vi "Encode Channels.vi"(8 "error in":errorcluster, 10 "Data and Parameters":T2 {"Data" format="%.0b"}, 11 "Values in":dbl[](array[numeric])) -> (0 "error out":errorcluster, 3 "Data":u8[](array[numeric]) format="%.0b")   [LabVIEW 2020, in "AIM ARINC 664 Engine.lvlib" / "Implementation.lvlib" / "Tx UDP Execution Unit.lvclass"]
uses:
  Tx UDP Execution Unit.lvclass
  <vilib>/NI/NI VeriStand Encoding and Decoding/Encoding.ctl
  b24d3698-aaae-4200-bf93-4b6af5480478.vi
  5b1080be-549e-4688-aad8-fb955257d8ef.vi
  b24d3698-aaae-4200-bf93-4b6af5480478.vi/9377bb8f-44b5-4a8f-87f1-966fd5a9edcc.vi
  b24d3698-aaae-4200-bf93-4b6af5480478.vi/e95d9d1f-307c-44d6-9f26-c3f519a4990d.vi
  b24d3698-aaae-4200-bf93-4b6af5480478.vi/0c23f515-4369-4514-bc3d-4444e6b437b2.vi
  5b1080be-549e-4688-aad8-fb955257d8ef.vi/136dcdcb-2dd3-4a4d-a796-a8f7a3f8e1ac.vi
  5b1080be-549e-4688-aad8-fb955257d8ef.vi/a54b505c-1216-4ef4-8378-3ceda9d188df.vi
  <vilib>/NI/NI VeriStand Encoding and Decoding/Get Bits Per Digit from Base.vi
  <vilib>/NI/NI VeriStand Encoding and Decoding/Encoding and Decoding.lvlib
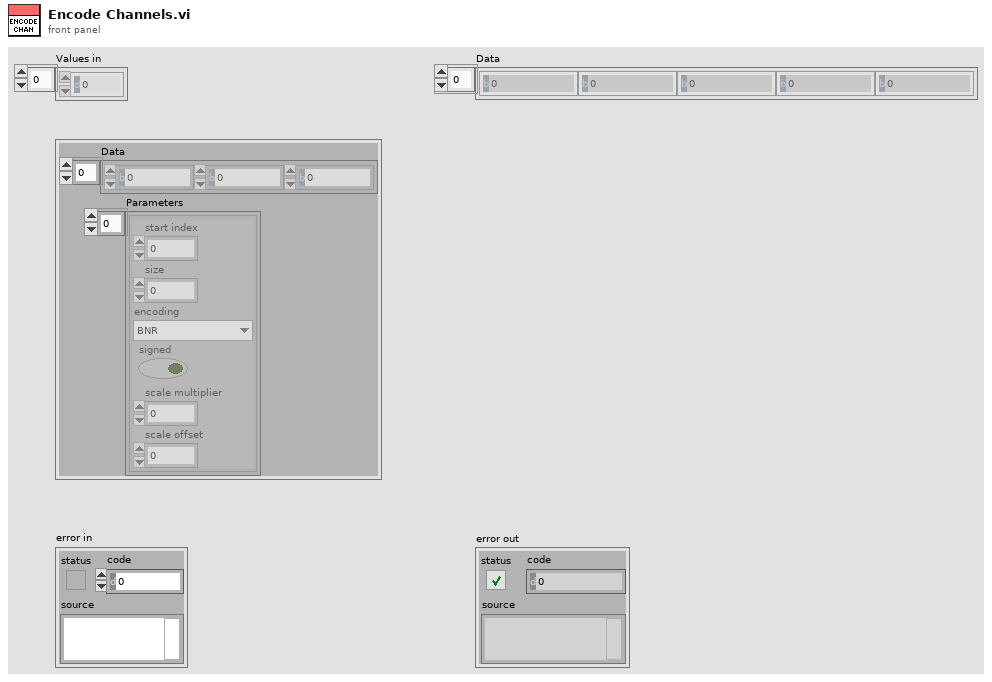
[diagram p1: front panel]
types:
  T1 = typedef "Encoding and Decoding.lvlib/Encoding.ctl" = enum16{"BNR", "BCD", "Discrete"}
  T2 = cluster{"Data":u8[], "Parameters":cluster{"start index":i32, "size":i32, "encoding":T1, "signed":bool, "scale multiplier":dbl, "scale offset":dbl}[]}
  T3 = cluster{"start index":i32, "size":i32, "encoding":T1, "signed":bool, "scale multiplier":dbl, "scale offset":dbl}[]
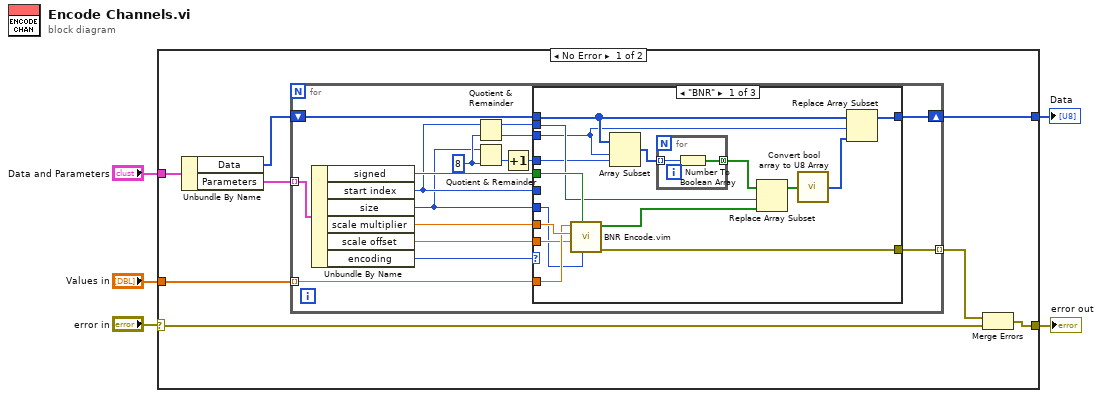
[diagram p0: block diagram]
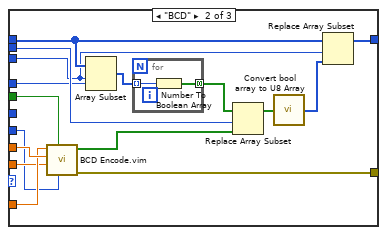
[diagram p2: hidden frame]
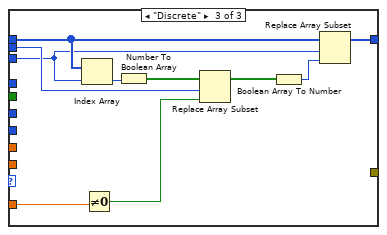
[diagram p3: hidden frame]
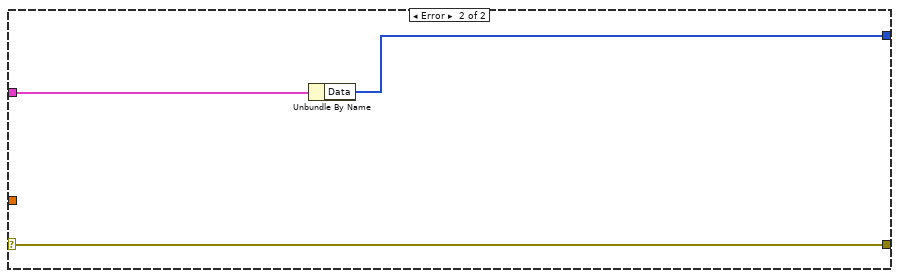
[diagram p4: hidden frame]
diagram:
  n1 = case shown="No Error" "error in" {
    selector: "error in" -> [w6 w78]
    tunnel: "Data and Parameters" -> [w13 w77]
    tunnel: "Values in" -> [w12 _]
    tunnel: [w9 w76] -> w3
    tunnel: [w7 w78] -> w1
    frame No Error {
      n2 = Unbundle By Name(w13) -> ("Data"=w10:u8[], "Parameters"=w11:T3)
      n3 = for {
        tunnel: w12 -> [w23] mode=indexing
        tunnel: w11 -> [w24] mode=indexing
        shift-right: [w19] -> w9
        shift-left: w10 -> [w26]
        tunnel: [w14] -> w8 mode=indexing
        w21 = 8 ("y")
        n4 = Unbundle By Name(w24) -> ("signed"=w25:bool, "start index"=w22:i32, "size"=w20:i32, "scale multiplier"=w28:dbl, "scale offset"=w27:dbl, "encoding"=w29:T1)
        n5 = Quotient & Remainder(x=w22, y=w21) -> (x-y*floor(x/y)=w17:i32, floor(x/y)=w18:i32)
        n6 = Quotient & Remainder(x=w20, y=w21) -> (floor(x/y)=w16:i32)  [unwired: 1 out]
        n7 = Increment(x=w16) -> (x+1=w15:i32)
        n8 = case shown="\"BNR\"" w29 {
          tunnel: w25 -> [w45 w63 _]
          tunnel: w28 -> [w44 w62 _]
          tunnel: w27 -> [w42 w60 _]
          tunnel: w26 -> [w40 w58 w75]
          tunnel: w22 -> [_ _ _]
          tunnel: w20 -> [w41 w59 _]
          tunnel: w23 -> [w43 w61 w70]
          tunnel: [w38 w56 w74] -> w19
          tunnel: w18 -> [w30 w48 w67]
          tunnel: w17 -> [w39 w57 w71]
          tunnel: w15 -> [w35 w53 _]
          tunnel: [w31 w49 _] -> w14
          frame "BNR" {
            n9 = call "BNR Encode.vim"("data size (bits)"=w41, "signed"=w45, "scale offset"=w42, "scale multiplier"=w44, "value"=w43) -> ("error out"=w31:errorcluster, "BNR encoded value"=w34:bool[])  [unwired: 5 in]
            n10 = Array Subset(array=w40, index=w30, length=w35) -> (w37:u8[])
            n11 = for {
              tunnel: w37 -> [w47] mode=indexing
              tunnel: [w46] -> w36 mode=concatenating
              n12 = Number To Boolean Array(number=w47) -> (Boolean array=w46:bool[])
            }
            n13 = Replace Array Subset(array=w36, new element=w34, index=w39) -> (w33:bool[])
            n14 = call "Convert bool array to U8 Array.vi"("Boolean array"=w33) -> ("Array"=w32:u8[])  [unwired: 14 in]
            n15 = Replace Array Subset(array=w40, new element=w32, index=w30) -> (w38:u8[])
          }
          frame "BCD" {
            n16 = call "BCD Encode.vim"("data size (bits)"=w59, "signed"=w63, "scale offset"=w60, "scale multiplier"=w62, "value"=w61) -> ("error out"=w49:errorcluster, "BCD encoded value"=w52:bool[])  [unwired: 4 in, 1 out]
            n17 = Array Subset(array=w58, index=w48, length=w53) -> (w55:u8[])
            n18 = for {
              tunnel: w55 -> [w65] mode=indexing
              tunnel: [w64] -> w54 mode=concatenating
              n19 = Number To Boolean Array(number=w65) -> (Boolean array=w64:bool[])
            }
            n20 = Replace Array Subset(array=w54, new element=w52, index=w57) -> (w51:bool[])
            n21 = call "Convert bool array to U8 Array.vi"("Boolean array"=w51) -> ("Array"=w50:u8[])  [unwired: 14 in]
            n22 = Replace Array Subset(array=w58, new element=w50, index=w48) -> (w56:u8[])
          }
          frame "Discrete" {
            n23 = Index Array(array=w75, index=w67) -> (element=w73:u8)
            n24 = Not Equal To 0?(x=w70) -> (x != 0?=w69:bool)
            n25 = Number To Boolean Array(number=w73) -> (Boolean array=w72:bool[])
            n26 = Replace Array Subset(array=w72, new element=w69, index=w71) -> (w68:bool[])
            n27 = Boolean Array To Number(Boolean array=w68) -> (number=w66:u32)
            n28 = Replace Array Subset(array=w75, new element=w66, index=w67) -> (w74:u8[])
          }
        }
      }
      n29 = Merge Errors(w8, w6) -> (w7:errorcluster)
    }
    frame Error {
      n30 = Unbundle By Name(w77) -> ("Data"=w76:u8[])
    }
  }
  "Data" <- w3
  "error out" <- w1
